vi "ParsePhasors.vi"(8 "error in (no error)":errorcluster, 9 "TimeStamp":ext format="%.4f", 10 "PktData":u8[](array[numeric]) format="%x", 11 "C37.118 PMU in":refnum<class "C37.118 PMU.lvclass">) -> (0 "error out":errorcluster, 2 "PmuReport":T1 {"Synx" format="%#_4g"; "Timestamp" format="%.6f"}, 3 "C37.118 PMU out":refnum<class "C37.118 PMU.lvclass">)   [LabVIEW 2018, in "SensorPlugins.lvlib" / "C37.118 PMU.lvclass"]
uses:
  C37.118 PMU.lvclass
  PmuBaseClass/Typedef/PmuData.ctl
  C37.118 PMU.lvclass/C37.118 PMU.ctl
  Accessors/Read PMUConfigData.vi
  PmuBaseClass/PmuBase.lvclass
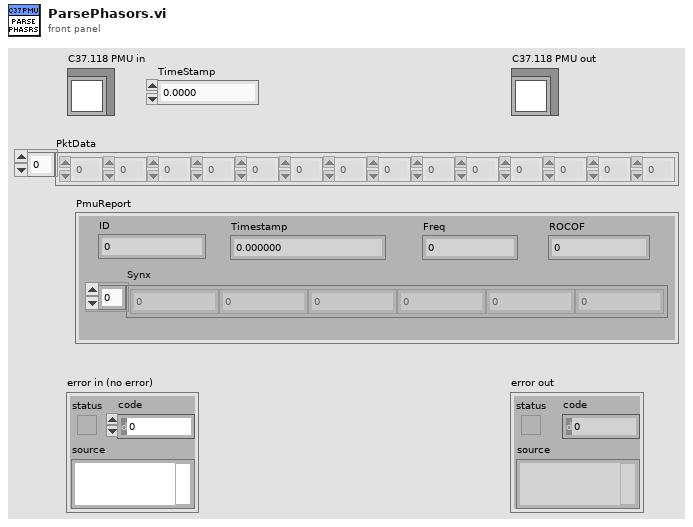
[diagram p1: front panel]
types:
  T1 = typedef "SensorPlugins.lvlib/PmuBase.lvclass/PmuData.ctl" = cluster{"Timestamp":dbl, "Synx":cdb[], "Freq":dbl, "ROCOF":dbl, "ID":i16}
  T2 = typedef "SensorPlugins.lvlib/C37.118 PMU.lvclass/PMUConfigData.ctl" = cluster{"TimeBase":u32, "NUM_PMU":u16, "Station Name":string, "IDCODE":u16, "PHRNMR":u16, "ANNMR":u16, "DIGNMR":u16, "FORMAT BITS":T3, "Valid Inputs":u16[], "DigitalStatusMask":u16[], "24bit_PHUNIT":i32[], "24bit_ANUNIT":u32[], "Analog Amplitude Setting":u32[], "Unit (Vor I)":u8[], "ChannelNames":string, "Fs":i16, "SOC ":u32, "FRACSEC":u32, "F0":sgl, "CFGCNT":u16}
  T3 = typedef "SensorPlugins.lvlib/C37.118 PMU.lvclass/FormatBits.ctl" = cluster{"Rect/Polar":bool, "Phasor Int/Float":bool, "Analog Int/Float":bool, "F/ROCOF Int/Float":bool}
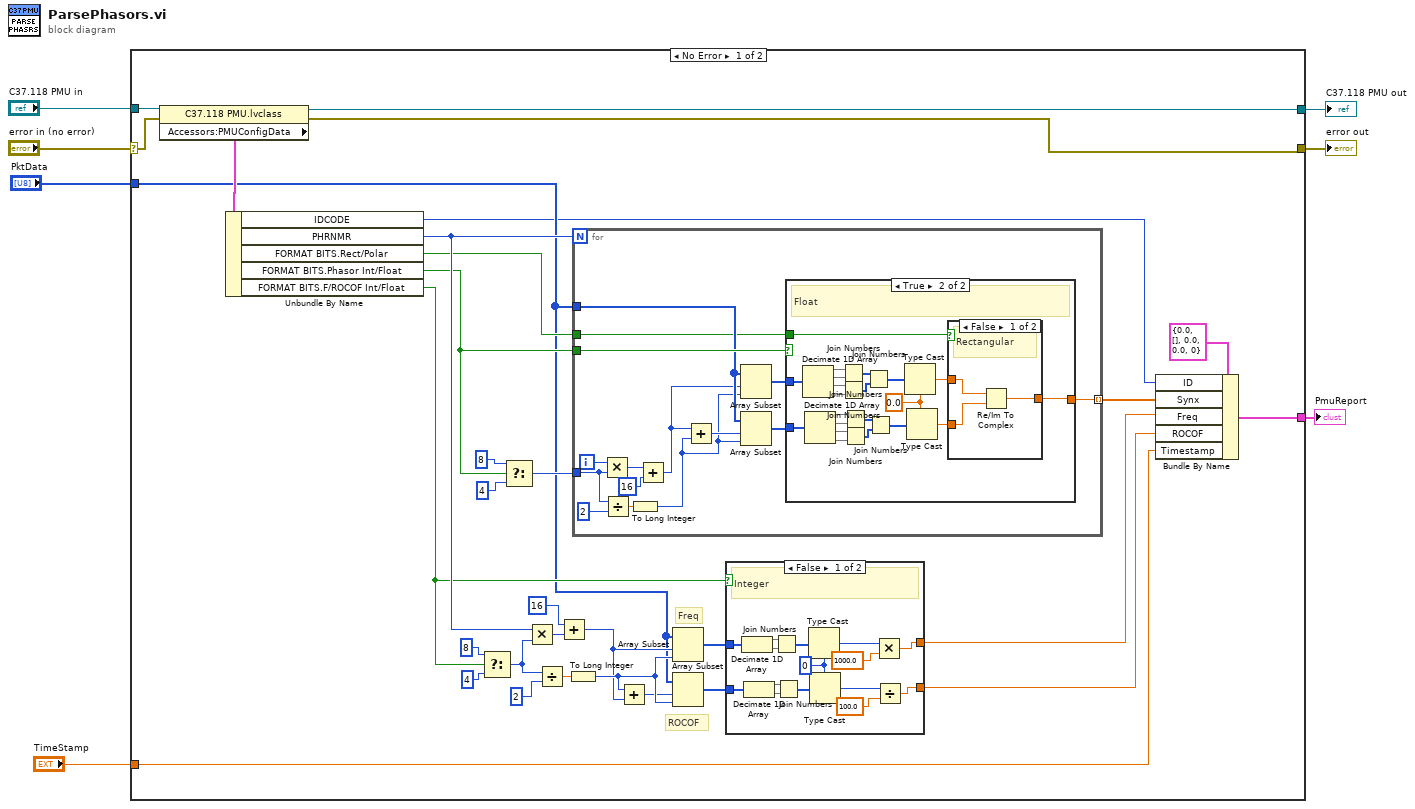
[diagram p0: block diagram]
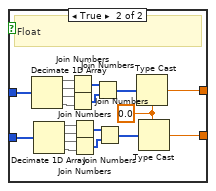
[diagram p2: hidden frame]
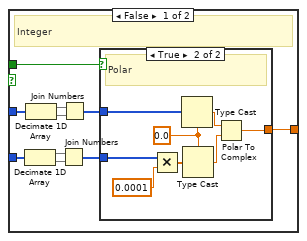
[diagram p3: hidden frame]
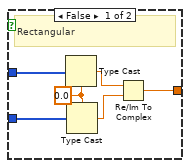
[diagram p4: hidden frame]
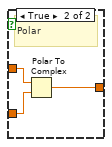
[diagram p5: hidden frame]
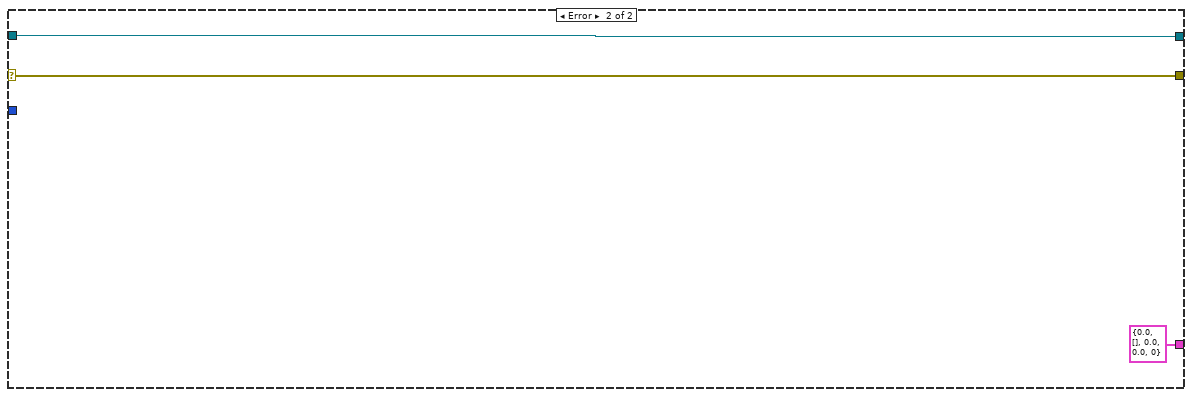
[diagram p6: hidden frame]
diagram:
  n1 = case shown="No Error" "error in (no error)" {
    selector: "error in (no error)" -> [w17 w142]
    tunnel: [w16 w142] -> w6
    tunnel: [w8 w141] -> w4
    tunnel: "C37.118 PMU in" -> [w24 w141]
    tunnel: "PktData" -> [w18 _]
    tunnel: "TimeStamp" -> [w10 _]
    tunnel: [w9 T1 {"Timestamp"=0.0, "Synx"=[], "Freq"=0.0, "ROCOF"=0.0, "ID"=0} ("PmuReport")] -> w1
    frame No Error {
      # "ROCOF"
      # "Freq"
      n2 = property class="C37.118 PMU.lvclass"(reference=w24, error in=w17) -> (reference out=w8:refnum<class "C37.118 PMU.lvclass">, error out=w16:errorcluster, "Accessors:PMUConfigData"=w23:T2)
      n3 = Unbundle By Name(w23) -> ("IDCODE"=w14:u16, "PHRNMR"=w22:u16, "FORMAT BITS.Rect/Polar"=w21:bool, "FORMAT BITS.Phasor Int/Float"=w20:bool, "FORMAT BITS.F/ROCOF Int/Float"=w19:bool)
      n4 = Select(t=8, s=w19, f=4) -> (s? t:f=w32:i32)
      n5 = Select(t=8, s=w20, f=4) -> (s? t:f=w37:i32)
      n6 = Multiply(x=w22, y=w32) -> (x*y=w34:i32)
      n7 = Divide(x=w32, y=2) -> (x/y=w31:dbl)
      n8 = Add(x=16, y=w34) -> (x+y=w27:i32)
      n9 = To Long Integer(number=w31) -> (32bit integer=w30:i32)
      n10 = for {
        N: w22 -> [_]
        tunnel: w20 -> [w88]
        tunnel: w37 -> [w86]
        tunnel: w18 -> [w81]
        tunnel: w21 -> [w78]
        tunnel: [w77] -> w13 mode=indexing
        i -> [w85]
        n11 = Multiply(x=w85, y=w86) -> (x*y=w84:i32)
        n12 = Divide(x=w86, y=2) -> (x/y=w83:dbl)
        n13 = To Long Integer(number=w83) -> (32bit integer=w74:i32)
        n14 = Add(x=w84, y=16 ("value")) -> (x+y=w75:i32)
        n15 = Add(x=w75, y=w74) -> (x+y=w82:i32)
        n16 = Array Subset(array=w81, index=w75, length=w74) -> (w80:u8[])
        n17 = Array Subset(array=w81, index=w82, length=w74) -> (w79:u8[])
        n18 = case shown="True" w88 {
          tunnel: w80 -> [w98 w133]
          tunnel: w79 -> [w97 w132]
          tunnel: w78 -> [w92 w116]
          tunnel: [w89 w113] -> w77
          frame False {
            # "Integer"
            n19 = Decimate 1D Array(w97) -> (w93:u8[], w94:u8[])
            n20 = Decimate 1D Array(w98) -> (w96:u8[], w95:u8[])
            n21 = Join Numbers(hi=w93, lo=w94) -> ((hi.lo)=w90:u16[])
            n22 = Join Numbers(hi=w96, lo=w95) -> ((hi.lo)=w91:u16[])
            n23 = case shown="True" w92 {
              tunnel: w91 -> [w104 w110]
              tunnel: w90 -> [w103 w112]
              tunnel: [w99 w105] -> w89
              frame False {
                w102 = sgl 0.0
                # "Rectangular"
                n24 = Type Cast(type=w102, x=w104) -> (*(type *) &x=w101:sgl)
                n25 = Type Cast(type=w102, x=w103) -> (*(type *) &x=w100:sgl)
                n26 = Re/Im To Complex(1:w100, 2:w101) -> (0:w99:csg)
              }
              frame True {
                w108 = sgl 0.0
                # "Polar"
                n27 = Multiply(x=w112, y=0.0001) -> (x*y=w109:dbl[])
                n28 = Type Cast(type=w108, x=w110) -> (*(type *) &x=w106:sgl)
                n29 = Type Cast(type=w108, x=w109) -> (*(type *) &x=w107:sgl)
                n30 = Polar To Complex(1:w107, 2:w106) -> (0:w105:csg)
              }
            }
          }
          frame True {
            w117 = sgl 0.0
            # "Float"
            n31 = Decimate 1D Array(w133) -> (w131:u8[], w130:u8[], w129:u8[], w128:u8[])
            n32 = Decimate 1D Array(w132) -> (w122:u8[], w121:u8[], w123:u8[], w120:u8[])
            n33 = Join Numbers(hi=w131, lo=w130) -> ((hi.lo)=w126:u16[])
            n34 = Join Numbers(hi=w129, lo=w128) -> ((hi.lo)=w127:u16[])
            n35 = Join Numbers(hi=w122, lo=w121) -> ((hi.lo)=w125:u16[])
            n36 = Join Numbers(hi=w123, lo=w120) -> ((hi.lo)=w124:u16[])
            n37 = Join Numbers(hi=w126, lo=w127) -> ((hi.lo)=w119:u32[])
            n38 = Join Numbers(hi=w125, lo=w124) -> ((hi.lo)=w118:u32[])
            n39 = Type Cast(type=w117, x=w119) -> (*(type *) &x=w115:sgl)
            n40 = Type Cast(type=w117, x=w118) -> (*(type *) &x=w114:sgl)
            n41 = case shown="False" w116 {
              tunnel: w115 -> [w135 w139]
              tunnel: w114 -> [w134 w138]
              tunnel: [w136 w137] -> w113
              frame False {
                # "Rectangular"
                n42 = Re/Im To Complex(1:w134, 2:w135) -> (0:w136:csg)
              }
              frame True {
                # "Polar"
                n43 = Polar To Complex(1:w138, 2:w139) -> (0:w137:csg)
              }
            }
          }
        }
      }
      n44 = Add(x=w30, y=w27) -> (x+y=w28:i32)
      n45 = Array Subset(array=w18, index=w27, length=w30) -> (w26:u8[])
      n46 = Array Subset(array=w18, index=w28, length=w30) -> (w25:u8[])
      n47 = case shown="False" w19 {
        tunnel: w26 -> [w54 w67]
        tunnel: w25 -> [w53 w60]
        tunnel: [w41 w56] -> w12
        tunnel: [w40 w55] -> w11
        frame False {
          w46 = i16 0
          # "Integer"
          n48 = Decimate 1D Array(w54) -> (w51:u8[], w52:u8[])
          n49 = Decimate 1D Array(w53) -> (w49:u8[], w50:u8[])
          n50 = Join Numbers(hi=w51, lo=w52) -> ((hi.lo)=w48:u16[])
          n51 = Join Numbers(hi=w49, lo=w50) -> ((hi.lo)=w47:u16[])
          n52 = Type Cast(type=w46, x=w48) -> (*(type *) &x=w45:i16)
          n53 = Type Cast(type=w46, x=w47) -> (*(type *) &x=w43:i16)
          n54 = Multiply(x=w45, y=sgl 1000.0) -> (x*y=w41:sgl)
          n55 = Divide(x=w43, y=sgl 100.0) -> (x/y=w40:sgl)
        }
        frame True {
          w59 = sgl 0.0
          # "Float"
          n56 = Decimate 1D Array(w67) -> (w68:u8[], w69:u8[], w70:u8[], w71:u8[])
          n57 = Decimate 1D Array(w60) -> (w66:u8[], w65:u8[], w64:u8[], w63:u8[])
          n58 = Join Numbers(hi=w68, lo=w69) -> ((hi.lo)=w73:u16[])
          n59 = Join Numbers(hi=w70, lo=w71) -> ((hi.lo)=w72:u16[])
          n60 = Join Numbers(hi=w66, lo=w65) -> ((hi.lo)=w61:u16[])
          n61 = Join Numbers(hi=w64, lo=w63) -> ((hi.lo)=w62:u16[])
          n62 = Join Numbers(hi=w73, lo=w72) -> ((hi.lo)=w57:u32[])
          n63 = Join Numbers(hi=w61, lo=w62) -> ((hi.lo)=w58:u32[])
          n64 = Type Cast(type=w59, x=w57) -> (*(type *) &x=w56:sgl)
          n65 = Type Cast(type=w59, x=w58) -> (*(type *) &x=w55:sgl)
        }
      }
      n66 = Bundle By Name(cluster=T1 {"Timestamp"=0.0, "Synx"=[], "Freq"=0.0, "ROCOF"=0.0, "ID"=0} ("PmuReport"), "ID"=w14, "Synx"=w13, "Freq"=w12, "ROCOF"=w11, "Timestamp"=w10) -> (w9:T1)
    }
    frame Error {
    }
  }
  "error out" <- w6
  "C37.118 PMU out" <- w4
  "PmuReport" <- w1
